vi "Verify_Upper and Lower Limit.vi"(0 "Upper Limits":dbl[](array[numeric]), 1 "R_Upper Limits":dbl[](array[numeric]), 2 "Array of Names":string[](array[string]), 3 "R_Array of Names":string[](array[string]), 5 "Lower Limits":dbl[](array[numeric]), 7 "Results":dbl[](array[numeric]), 11 "Error In":errorcluster, 12 "R_Results":dbl[](array[numeric]), 13 "R_Lower Limits":dbl[](array[numeric])) -> (4 "Pass/Fail?":bool, 6 "Report Text":string, 8 "Pass/Fail Array":bool[](array[boolean]), 15 "Error Out":errorcluster)   [LabVIEW 2016, in "2015 VA Washer.lvlib"]
uses:
  Projects/2015 VA Washer.lvlib
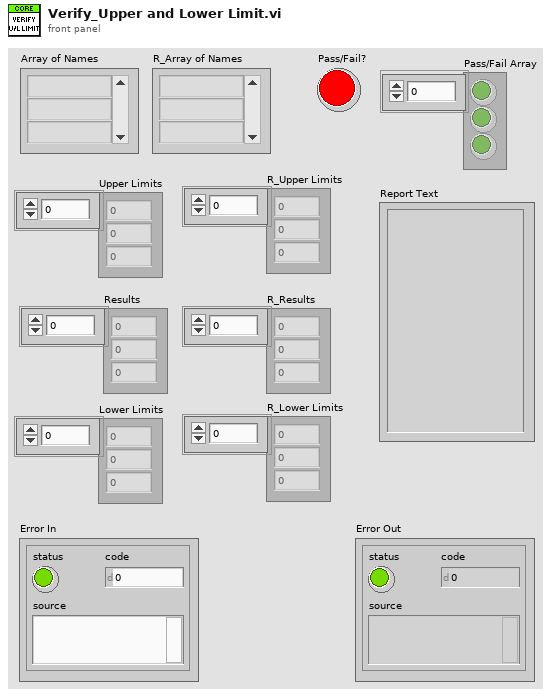
[diagram p1: front panel]
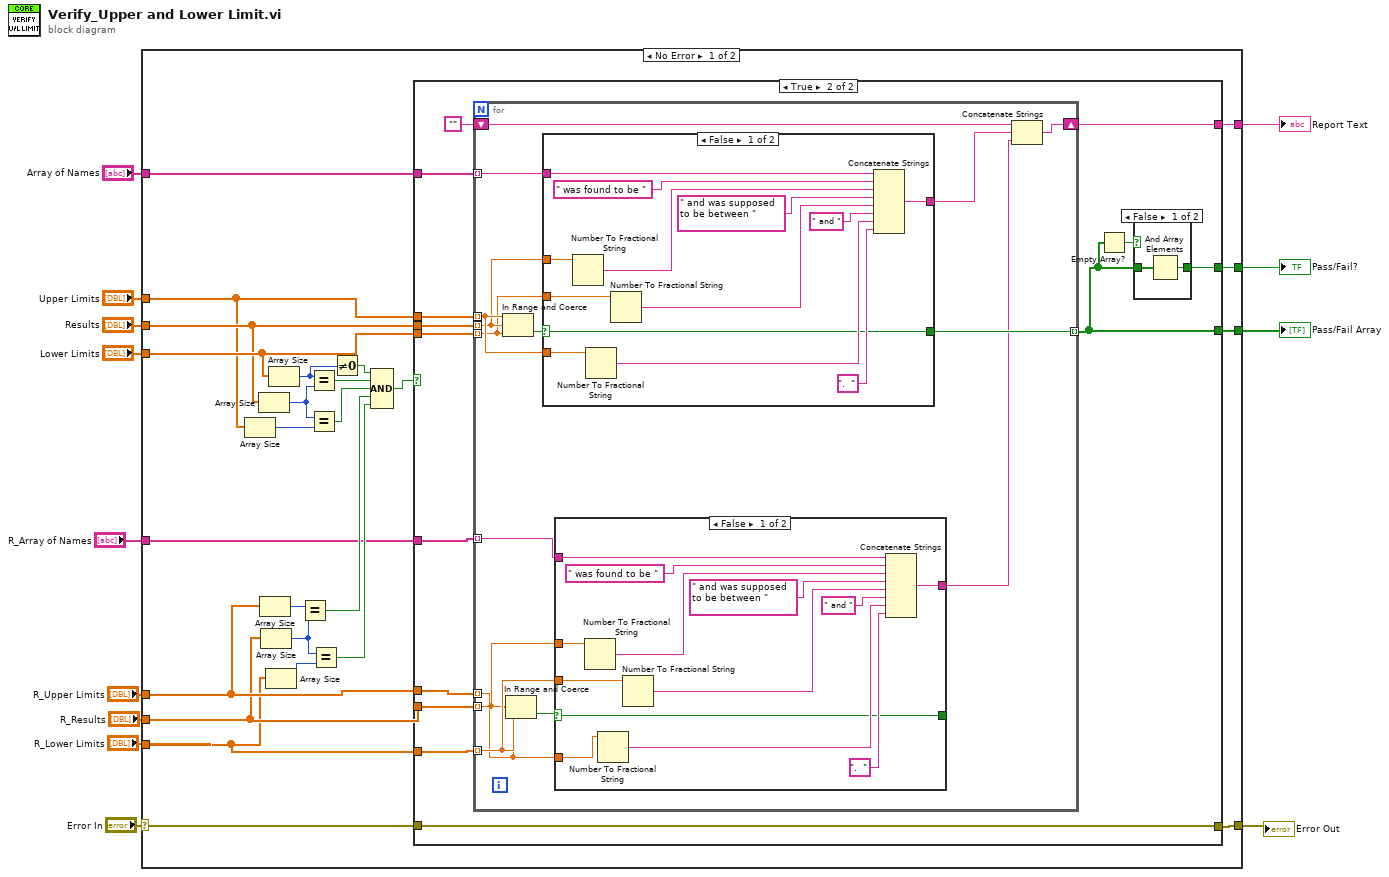
[diagram p0: block diagram]
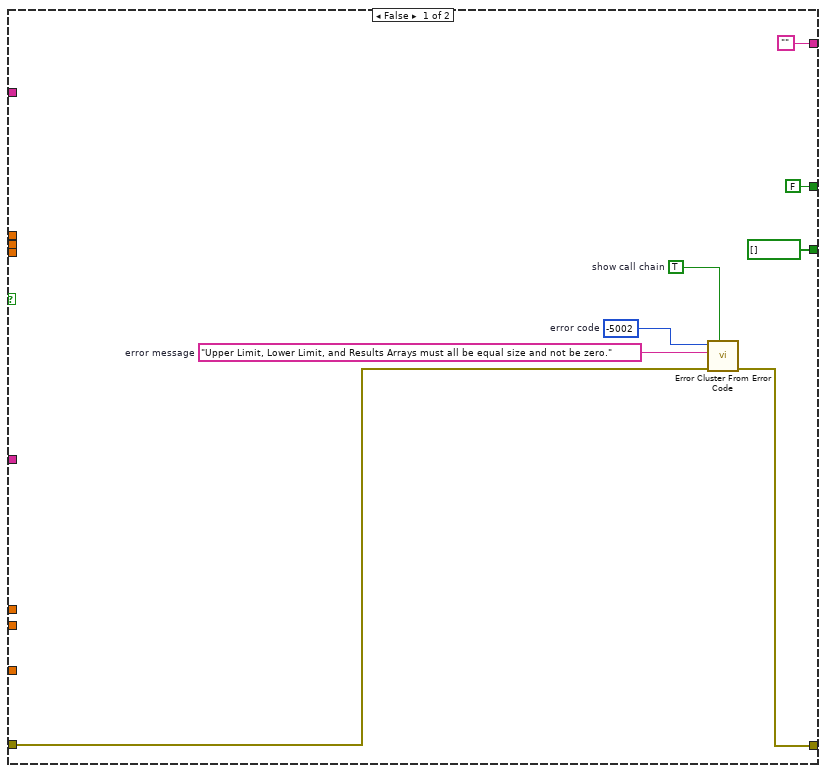
[diagram p2: hidden frame]
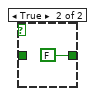
[diagram p3: hidden frame]
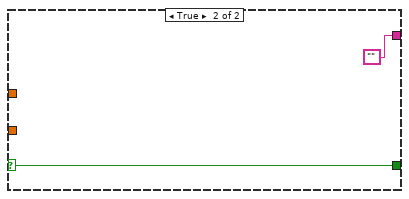
[diagram p4: hidden frame]
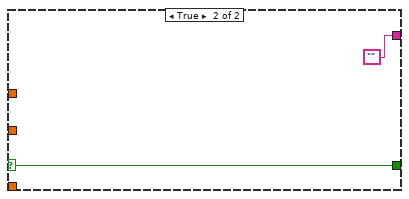
[diagram p5: hidden frame]
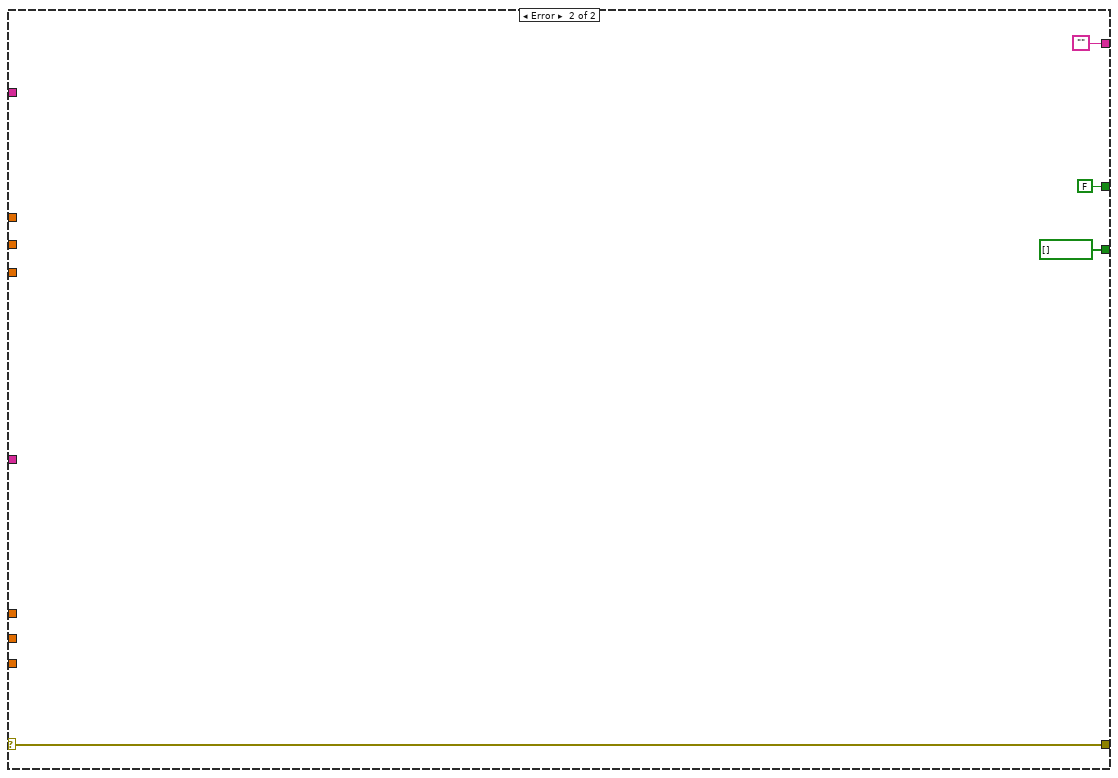
[diagram p6: hidden frame]
diagram:
  n1 = case shown="No Error" "Error In" {
    selector: "Error In" -> [w23 w112]
    tunnel: [w38 ""] -> w13
    tunnel: "Upper Limits" -> [w32 _]
    tunnel: "Lower Limits" -> [w34 _]
    tunnel: "Results" -> [w33 _]
    tunnel: "Array of Names" -> [w37 _]
    tunnel: [w36 bool[] []] -> w9
    tunnel: [w35 FALSE] -> w8
    tunnel: [w24 w112] -> w6
    tunnel: "R_Upper Limits" -> [w17 _]
    tunnel: "R_Results" -> [w16 _]
    tunnel: "R_Lower Limits" -> [w15 _]
    tunnel: "R_Array of Names" -> [w14 _]
    frame No Error {
      n2 = Array Size(array=w32) -> (size(s)=w31:i32)
      n3 = Array Size(array=w33) -> (size(s)=w30:i32)
      n4 = Array Size(array=w17) -> (size(s)=w21:i32)
      n5 = Array Size(array=w16) -> (size(s)=w22:i32)
      n6 = Array Size(array=w15) -> (size(s)=w20:i32)
      n7 = Array Size(array=w34) -> (size(s)=w29:i32)
      n8 = Equal?(x=w21, y=w22) -> (x = y?=w19:bool)
      n9 = Equal?(x=w29, y=w30) -> (x = y?=w27:bool)
      n10 = Equal?(x=w30, y=w31) -> (x = y?=w26:bool)
      n11 = Equal?(x=w22, y=w20) -> (x = y?=w18:bool)
      n12 = Not Equal To 0?(x=w29) -> (x != 0?=w28:bool)
      n13 = Compound Arithmetic op=AND(w28, w27, w26, w19, w18) -> (w25:bool)
      n14 = case shown="True" w25 {
        tunnel: ["" w60] -> w38
        tunnel: w37 -> [_ w58]
        tunnel: [bool[] [] w56] -> w36
        tunnel: [FALSE w55] -> w35
        tunnel: w34 -> [_ w54]
        tunnel: w33 -> [_ w53]
        tunnel: w32 -> [_ w52]
        tunnel: w23 -> [w46 w51]
        tunnel: [w45 w51] -> w24
        tunnel: w17 -> [_ w48]
        tunnel: w16 -> [_ w50]
        tunnel: w15 -> [_ w49]
        tunnel: w14 -> [_ w47]
        frame False {
          w42 = "Upper Limit, Lower Limit, and Results Arrays must all be equal size and not be zero."  # error message
          w43 = -5002  # error code
          w44 = TRUE  # show call chain
          n15 = call <vilib>:"Error Cluster From Error Code.vi"("show call chain? (False)"=w44, "error in (no error)"=w46, "error message (\"\")"=w42, "error code (0)"=w43) -> ("error out"=w45:errorcluster)  [unwired: 5 in]
        }
        frame True {
          n16 = for {
            tunnel: w53 -> [w76] mode=indexing
            tunnel: w54 -> [w75] mode=indexing
            tunnel: w52 -> [w77] mode=indexing
            tunnel: [w74] -> w56 mode=indexing
            shift-right: [w72] -> w60
            shift-left: "" -> [w71]
            tunnel: w58 -> [w70] mode=indexing
            tunnel: w48 -> [w67] mode=indexing
            tunnel: w50 -> [w68] mode=indexing
            tunnel: w49 -> [w69] mode=indexing
            tunnel: w47 -> [w64] mode=indexing
            n17 = In Range and Coerce(upper limit=w77, x=w76, lower limit=w75) -> (In Range?=w78:bool)  [unwired: 1 out]
            n18 = In Range and Coerce(upper limit=w67, x=w68, lower limit=w69) -> (In Range?=w65:bool)  [unwired: 1 out]
            n19 = case shown="False" w78 {
              selector: w78 -> [w98 w108]
              tunnel: w77 -> [w95 _]
              tunnel: w76 -> [w106 _]
              tunnel: w75 -> [w96 _]
              tunnel: [w98 w108] -> w74
              tunnel: [w97 ""] -> w73
              tunnel: w70 -> [w94 _]
              frame False {
                n20 = Number To Fractional String(number=w106) -> (F-format string=w104:string)  [unwired: 3 in]
                n21 = Number To Fractional String(number=w95) -> (F-format string=w100:string)  [unwired: 3 in]
                n22 = Number To Fractional String(number=w96) -> (F-format string=w102:string)  [unwired: 3 in]
                n23 = Concatenate Strings(w94, " was found to be ", w104, " and was supposed to be between ", w102, " and " ("string"), w100, ".  " ("string")) -> (w97:string)
              }
              frame True {
              }
            }
            n24 = case shown="False" w65 {
              selector: w65 -> [w83 w93]
              tunnel: w68 -> [w91 _]
              tunnel: w69 -> [w81 _]
              tunnel: [w83 w93] -> _
              tunnel: [w82 ""] -> w66
              tunnel: w64 -> [w80 _]
              tunnel: w67 -> [w79 _]
              frame False {
                n25 = Number To Fractional String(number=w91) -> (F-format string=w89:string)  [unwired: 3 in]
                n26 = Number To Fractional String(number=w79) -> (F-format string=w85:string)  [unwired: 3 in]
                n27 = Number To Fractional String(number=w81) -> (F-format string=w87:string)  [unwired: 3 in]
                n28 = Concatenate Strings(w80, " was found to be ", w89, " and was supposed to be between ", w87, " and " ("string"), w85, ".  " ("string")) -> (w82:string)
              }
              frame True {
              }
            }
            n29 = Concatenate Strings(w71, w73, w66) -> (w72:string)
          }
          n30 = Empty Array?(array=w56) -> (empty?=w57:bool)
          n31 = case shown="False" w57 {
            tunnel: [w61 FALSE] -> w55
            tunnel: w56 -> [w62 _]
            frame False {
              n32 = And Array Elements(Boolean array=w62) -> (logical AND=w61:bool)
            }
            frame True {
            }
          }
        }
      }
    }
    frame Error {
    }
  }
  "Pass/Fail Array" <- w9
  "Report Text" <- w13
  "Pass/Fail?" <- w8
  "Error Out" <- w6
